vi "Intensity-XY2rPhi (SubVI).vi"(2 "Radius*Scale Factor":dbl, 3 "XY Array":dbl[][](array[numeric])) -> (0 "2D Array: r, phi, intensity":dbl[][](array[numeric]), 1 "X,Y, intensity":dbl[][](array[numeric]))   [LabVIEW 2016]
uses:
  <vilib>/ptbypt/NI_PtbyPt.lvlib
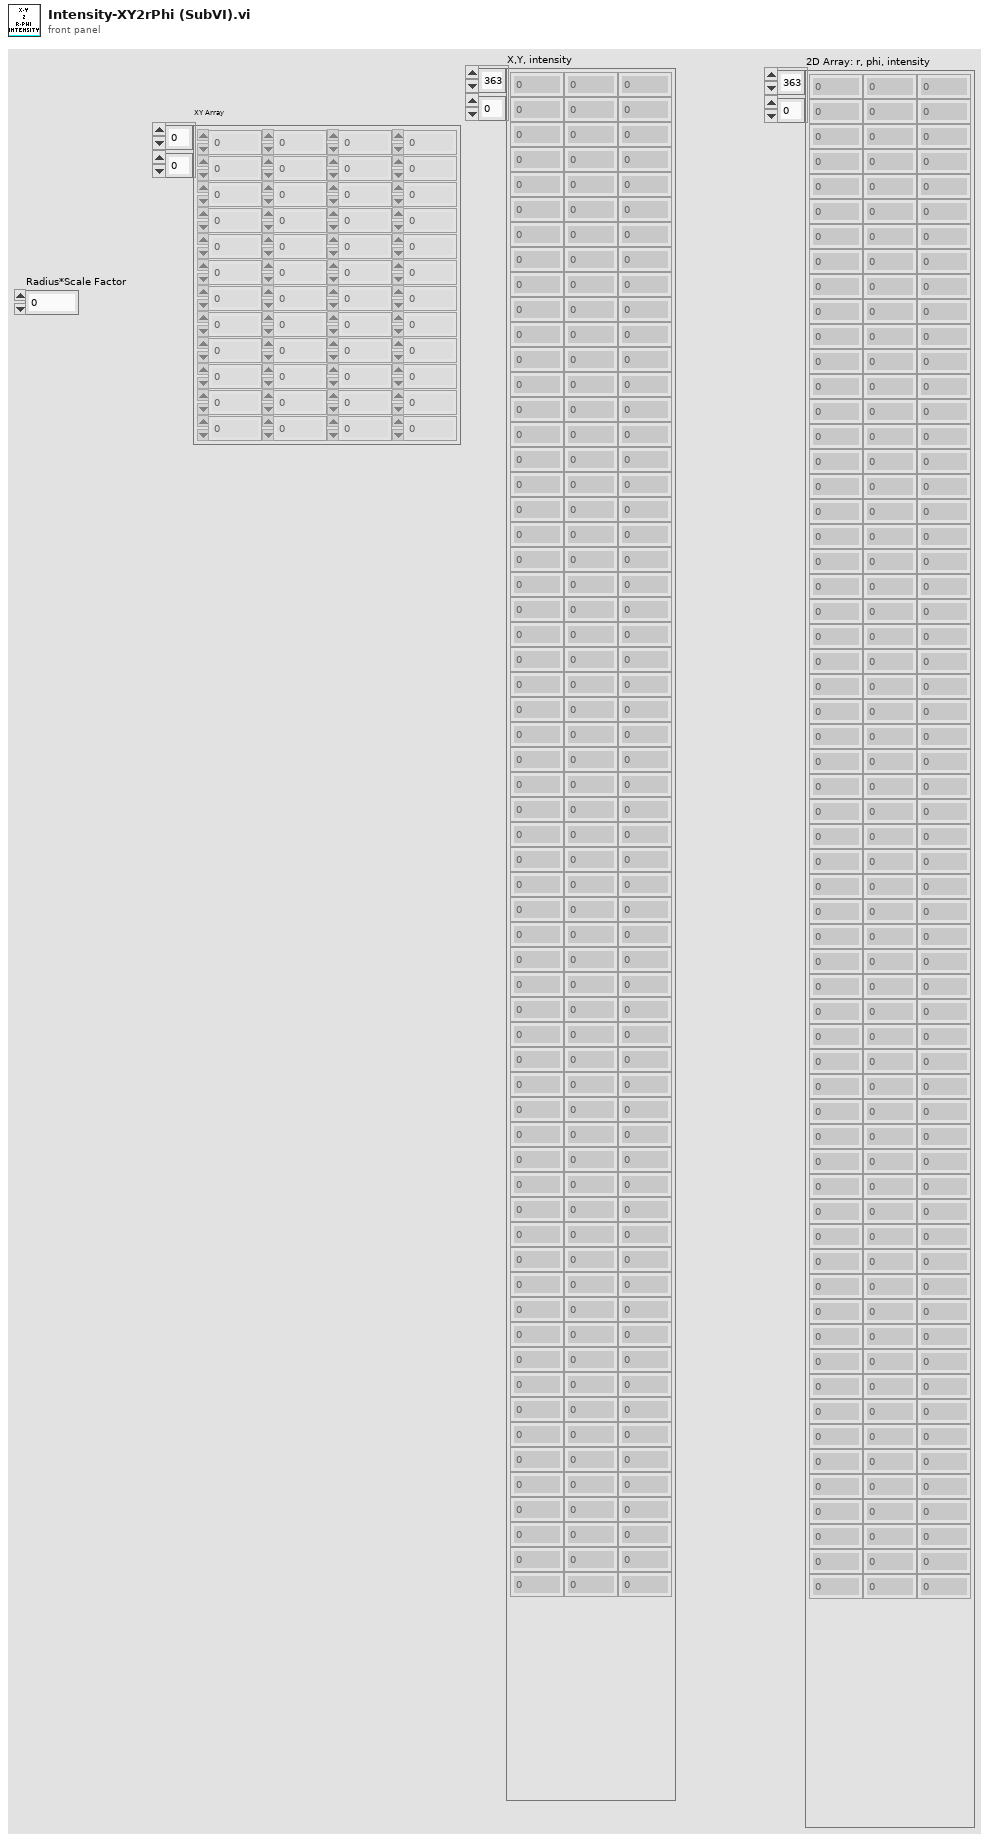
[diagram p1: front panel]
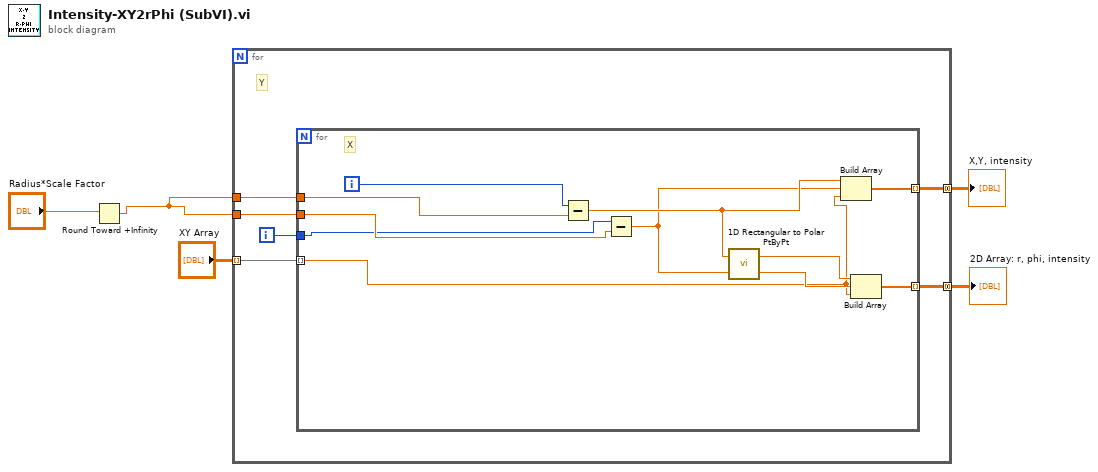
[diagram p0: block diagram]
diagram:
  n1 = Round Toward +Infinity(x="Radius*Scale Factor") -> (ceil(x): smallest int >= x=w1:dbl)
  n2 = for {
    tunnel: "XY Array" -> [w11] mode=indexing
    tunnel: [w9] -> w4 mode=concatenating
    tunnel: w1 -> [w8]
    tunnel: w1 -> [w7]
    tunnel: [w6] -> w3 mode=concatenating
    i -> [w10]
    # "Y"
    n3 = for {
      tunnel: w11 -> [w15] mode=indexing
      tunnel: [w21] -> w9 mode=indexing
      tunnel: w10 -> [w12]
      tunnel: w8 -> [w20]
      tunnel: w7 -> [w19]
      tunnel: [w14] -> w6 mode=indexing
      i -> [w13]
      # "X"
      n4 = Subtract(x=w13, y=w20) -> (x-y=w17:dbl)
      n5 = Subtract(x=w12, y=w19) -> (x-y=w16:dbl)
      n6 = call <vilib>:"1D Rectangular to Polar PtByPt.vi"("y"=w16, "x"=w17) -> ("phase"=w22:dbl, "magnitude"=w18:dbl)
      n7 = Build Array(w17, w16, w15) -> (w14:dbl[])
      n8 = Build Array(w18, w22, w15) -> (w21:dbl[])
    }
  }
  "2D Array: r, phi, intensity" <- w4
  "X,Y, intensity" <- w3
